vi "build auth URI.vi"(8 "error in (no error)":errorcluster, 10 "State Parameter":string, 11 "Oauth2 in":refnum<class "Oauth2.lvclass">) -> (0 "error out":errorcluster, 2 "Authorization Request URI":string, 3 "Oauth2":refnum<class "Oauth2.lvclass">)   [LabVIEW 2017, in "Oauth2.lvclass"]
uses:
  Oauth2.lvclass
  OAuthToken/OAuth2 Token Element -- enum.ctl
  Oauth2.lvclass/Oauth2.ctl
  <vilib>/LabVIEW Open Source Project/OpenURI/uri/URI.lvclass
  <vilib>/LabVIEW Open Source Project/Unicity/RandomStringGenerator/RandomStringGenerator.lvclass
  <vilib>/LabVIEW Open Source Project/OpenSerializer.Base64/Serializer.Base64.lvclass
  OAuthToken/OAuthAccessToken.lvclass
  <vilib>/LabVIEW Open Source Project/OpenURI/openURI.lvlib
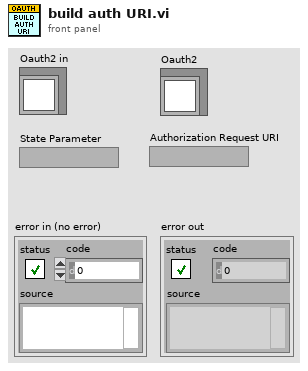
[diagram p1: front panel]
types:
  T1 = typedef "OAuthAccessToken.lvclass/OAuth2 Token Element -- enum.ctl" = enum16{"client_id", "client_secret", "response_type", "scope", "redirect_uri", "error", "error_description", "error_uri", "grant_type", "code", "access_token", "token_type", "expires_in", "username", "password", "refresh_token", "code_challenge", "code_challenge_method", "reverse_proxy_uri", "endpoint element", "prompt", "access_type", "id_token"}
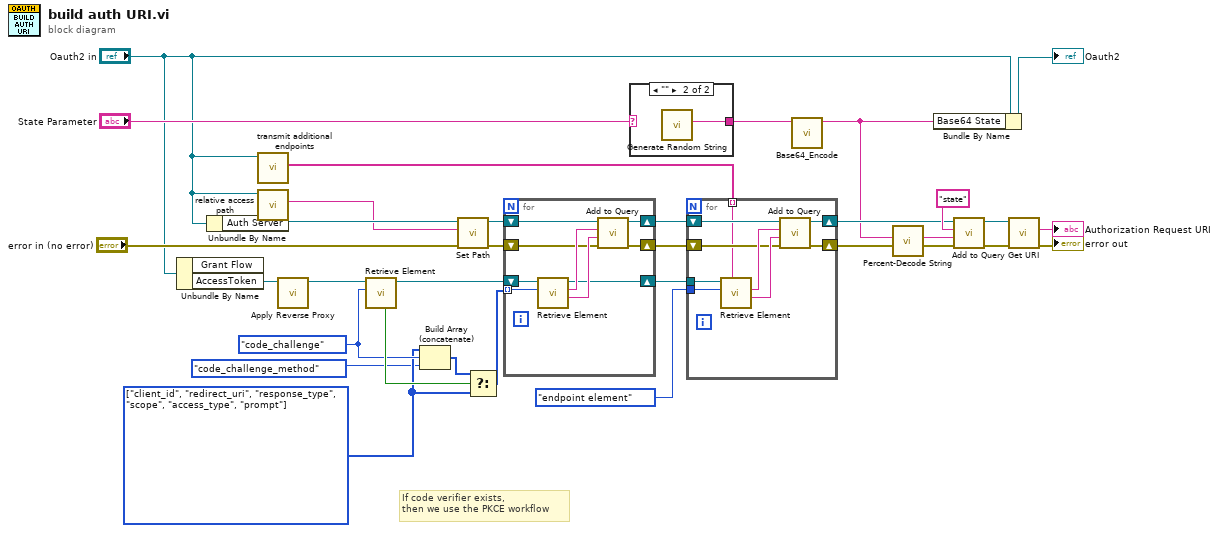
[diagram p0: block diagram]
diagram:
  w12 = OAuth2_Token_Element_--_enum."code_challenge" ("Token element")
  w10 = T1[] [enum."client_id", enum."redirect_uri", enum."response_type", enum."scope", enum."access_type", enum."prompt"] items=["client_id", "client_secret", "response_type", "scope", "redirect_uri", "error", "error_description", "error_uri", "grant_type", "code", "access_token", "token_type", "expires_in", "username", "password", "refresh_token", "code_challenge", "code_challenge_method", "reverse_proxy_uri", "endpoint element", "prompt", "access_type", "id_token"]
  # "If code verifier exists, \nthen we use the PKCE workflow"
  n1 = Unbundle By Name("Oauth2 in") -> ("AccessToken"=w3:refnum<class "OAuthAccessToken.lvclass">)  [unwired: 1 out]
  n2 = Unbundle By Name("Oauth2 in") -> ("Auth Server"=w29:refnum<class "URI.lvclass">)
  n3 = call-dynamic "transmit additional endpoints.vi"("Oauth2"="Oauth2 in") -> ("Additional Endpoints"=w19:string[])  [unwired: 10 in]
  n4 = call-dynamic "relative access path.vi"("Oauth2 in"="Oauth2 in") -> ("Authorization Path"=w1:string)  [unwired: 9 in, 1 out]
  n5 = call "Apply Reverse Proxy.vi"("OAuthAccessToken in"=w3) -> ("OAuthAccessToken out"=w2:refnum<class "OAuthAccessToken.lvclass">)  [unwired: 9 in, 1 out]
  n6 = call "Retrieve Element.vi"("Token element"=w12, "OAuthAccessToken in"=w2) -> ("OAuthAccessToken out"=w14:refnum<class "OAuthAccessToken.lvclass">, "element found"=w13:bool)  [unwired: 5 in, 3 out]
  n7 = Build Array (concatenate)(w10, w12, OAuth2_Token_Element_--_enum."code_challenge_method" ("Token element")) -> (w11:T1[])
  n8 = call <vilib>:"Set Path.vi"("error in (no error)"="error in (no error)", "path"=w1, "URI in"=w29) -> ("error out"=w24:errorcluster, "URI out"=w25:refnum<class "URI.lvclass">)  [unwired: 7 in]
  n9 = Select(t=w11, s=w13, f=w10) -> (s? t:f=w9:T1[])
  n10 = for {
    tunnel: w9 -> [w40] mode=indexing
    shift-right: [w38] -> w23
    shift-left: w25 -> [w39]
    shift-right: [w34] -> w21
    shift-left: w24 -> [w35]
    shift-right: [w33] -> w18
    shift-left: w14 -> [w41]
    n11 = call "Retrieve Element.vi"("Token element"=w40, "OAuthAccessToken in"=w41) -> ("Value"=w36:string, "Key"=w37:string, "OAuthAccessToken out"=w33:refnum<class "OAuthAccessToken.lvclass">)  [unwired: 5 in, 2 out]
    n12 = call <vilib>:"Add to Query.vi"("error in (no error)"=w35, "value"=w36, "key"=w37, "URI in"=w39) -> ("error out"=w34:errorcluster, "URI out"=w38:refnum<class "URI.lvclass">)  [unwired: 6 in]
  }
  n13 = case shown="\"\"" "State Parameter" {
    selector: "State Parameter" -> [w42 _]
    tunnel: [w42 w43] -> w27
    frame Default {
    }
    frame "" {
      n14 = call <vilib>:"Generate Random String.vi"() -> ("Random String"=w43:string)  [unwired: 11 in]
    }
  }
  n15 = for {
    tunnel: w18 -> [w52]
    shift-right: [w50] -> w22
    shift-left: w23 -> [w51]
    shift-right: [w46] -> w20
    shift-left: w21 -> [w47]
    tunnel: w19 -> [w44] mode=indexing
    tunnel: OAuth2_Token_Element_--_enum."endpoint element" ("Token element") -> [w45]
    n16 = call "Retrieve Element.vi"("Endpoint element key"=w44, "Token element"=w45, "OAuthAccessToken in"=w52) -> ("Value"=w48:string, "Key"=w49:string)  [unwired: 4 in, 3 out]
    n17 = call <vilib>:"Add to Query.vi"("error in (no error)"=w47, "value"=w48, "key"=w49, "URI in"=w51) -> ("error out"=w46:errorcluster, "URI out"=w50:refnum<class "URI.lvclass">)  [unwired: 6 in]
  }
  n18 = call <vilib>:"Base64_Encode.vi"("String"=w27) -> ("Encoded String"=w16:string)  [unwired: 9 in, 1 out]
  n19 = call <vilib>:"Percent-Decode String.vi"("Pct-Encoded String"=w16) -> ("String"=w15:string)  [unwired: 10 in]
  n20 = Bundle By Name(cluster="Oauth2 in", "Base64 State"=w16) -> (→"Oauth2":refnum<class "Oauth2.lvclass">)
  n21 = call <vilib>:"Add to Query.vi"("error in (no error)"=w20, "value"=w15, "key"="state" ("argument"), "URI in"=w22) -> ("error out"=w5:errorcluster, "URI out"=w6:refnum<class "URI.lvclass">)  [unwired: 6 in]
  n22 = call <vilib>:"Get URI.vi"("error in (no error)"=w5, "URI in"=w6) -> ("error out"=→"error out":errorcluster, "URI String"=→"Authorization Request URI":string)  [unwired: 7 in, 1 out]
